vi "Untitled 90.vi"   [LabVIEW 2012]
uses:
  <vilib>/NXT/Subs/MotorOutput.ctl
  <vilib>/NXT/Dual Mode Library/Waits/Wait_Num.vi
types:
  T1 = typedef "MotorOutput.ctl" = u8
  T2 = typedef "LVHSConnector.ctl" = cluster{"Hardware":string, "Flattened String":string}
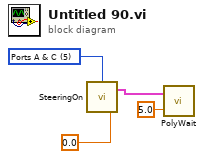
[diagram p0: block diagram]
diagram:
  w4 = T1 5 items=["Port A"=0, "Port B"=1, "Port C"=2, "Ports A & B"=4, "Ports A & C"=5, "Ports B & C"=6, "All Ports"=3] ("Output Ports (A & B)")
  n1 = call <vilib>:"SteeringOn.vi"("Steering (100)"=sgl 0.0 ("Time (1 sec)"), "Output Ports (A & B)"=w4) -> ("NXT"=w3:T2)  [unwired: 2 in]
  n2 = call-poly <vilib>:"PolyWait.vi"("Time (1 sec)"=sgl 5.0, "NXT"=w3) -> ()  [unwired: 2 in, 1 out]
